vi "Save To File (Digital Serial).vi"(8 "error in (no error)":errorcluster, 10 "digital serial input settings":T1={"number of channels"=51200, "data justification"=enum."Right Justified", "endianness"=enum."MSB First", "channel length"=0, "bit depth"=0, "frame clock rate"=0.0, "bit clock edge sync"=enum."Falling", "master clock source"=enum."Internal", "master clock rate"=0.0, "Logic Level"=enum."1.2 V", "frame sync edge for channel 0"=enum."Rising", "Channel 0 Offset"=0}, 11 "file path":path) -> (0 "error out":errorcluster)   [LabVIEW 2022 SP3, in "input cfg file.lvlib"]
uses:
  input cfg file.lvlib
  controls/digital serial audio/digital serial input settings.ctl
  <vilib>/PDM Acquisition Toolkit/shared/controls/PCM Data Justification.ctl
  <vilib>/PDM Acquisition Toolkit/shared/controls/PCM Bit Endianness.ctl
  <vilib>/PDM Acquisition Toolkit/shared/controls/Digital Edge.ctl
  controls/master clock source.ctl
  <vilib>/PDM Acquisition Toolkit/host/Classes/Session/Controls/Logic Levels.ctl
  controls/input type.ctl
  digital serial/digital serial input cfg file.lvlib
  <vilib>/PDM Acquisition Toolkit/shared/PDM Shared.lvlib
  <vilib>/PDM Acquisition Toolkit/host/Classes/Session/DecoderSession.lvclass
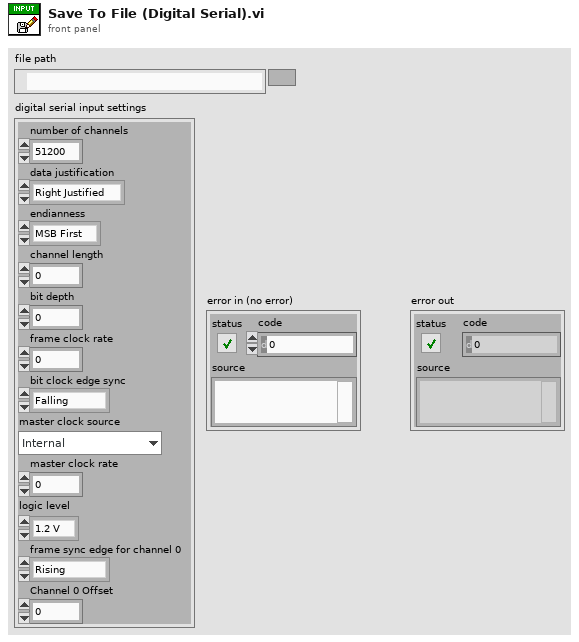
[diagram p1: front panel]
types:
  T1 = typedef "digital serial input settings.ctl" = cluster{"number of channels":u32, "data justification":T2, "endianness":T3, "channel length":u32, "bit depth":u32, "frame clock rate":dbl, "bit clock edge sync":T4, "master clock source":T5, "master clock rate":dbl, "Logic Level":T6, "frame sync edge for channel 0":T4, "Channel 0 Offset":u32}
  T2 = typedef "PDM Shared.lvlib/PCM Data Justification.ctl" = enum16{"Left Justified", "Right Justified"}
  T3 = typedef "PDM Shared.lvlib/PCM Bit Endianness.ctl" = enum16{"MSB First", "LSB First"}
  T4 = typedef "PDM Shared.lvlib/Digital Edge.ctl" = enum8{"Rising", "Falling"}
  T5 = typedef "master clock source.ctl" = enum32{"Internal", "External"}
  T6 = typedef "PDM Acquisition Class Library.lvlib/DecoderSession.lvclass/Logic Levels.ctl" = enum16{"3.3 V", "1.8 V", "1.2 V"}
  T7 = typedef "input type.ctl" = enum32{"Digital Serial", "PDM"}
  T8 = typedef "digital serial input settings_json.ctl" = cluster{"number of channels":u32, "data justification":string, "endianness":string, "channel length":u32, "bit depth":u32, "frame clock rate":dbl, "bit clock edge sync":string, "master clock souce":string, "master clock rate":dbl, "logic level":string, "frame sync edge for channel 0":string, "Channel 0 Offset":u32}
  T9 = enum16{"open", "replace", "create", "open or create", "replace or create", "replace or create with confirmation"}
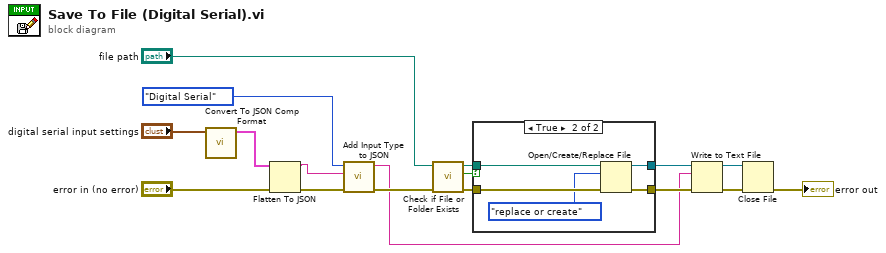
[diagram p0: block diagram]
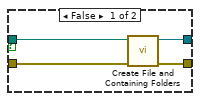
[diagram p2: hidden frame]
diagram:
  n1 = call "Convert To JSON Comp Format.vi"("input settings"="digital serial input settings") -> ("input settings JSON"=w1:cluster{"digital serial":T8})  [unwired: 10 in]
  n2 = Flatten To JSON(anything=w1, error in (no error)="error in (no error)") -> (JSON string=w5:string, 11:w7:errorcluster)  [unwired: 1 in]
  n3 = call "Add Input Type to JSON.vi"("error in (no error)"=w7, "input cfg JSON"=w5, "input type"=input_type."Digital Serial") -> ("error out"=w6:errorcluster, "input cfg JSON"=w4:string)  [unwired: 7 in]
  n4 = call <vilib>:"Check if File or Folder Exists.vi"("error in (no error)"=w6, "path"="file path") -> ("error out"=w10:errorcluster, "file or folder exists?"=w9:bool, "dup path"=w8:path)  [unwired: 7 in]
  n5 = case shown="True" w9 {
    tunnel: [w21 w26] -> w16
    tunnel: [w20 w23] -> w15
    tunnel: w10 -> [w19 w24]
    tunnel: w8 -> [w18 w25]
    frame False {
      n6 = call <vilib>:"Create File and Containing Folders.vi"("error in (no error)"=w19, "file path"=w18) -> ("error out"=w21:errorcluster, "refnum out"=w20:refnum<file>)  [unwired: 8 in]
    }
    frame True {
      n7 = Open/Create/Replace File(file path (use dialog)=w25, error in=w24, operation (0:open)=T9."replace or create") -> (refnum out=w23:refnum<file>, error out=w26:errorcluster)  [unwired: 3 in, 1 out]
    }
  }
  n8 = Write to Text File(file (use dialog)=w15, text=w4, error in=w16) -> (refnum out=w13:refnum<file>, error out=w14:errorcluster)  [unwired: 1 in, 1 out]
  n9 = Close File(refnum=w13, error in=w14) -> (error out=→"error out":errorcluster)  [unwired: 1 out]
